vi "Color-Senser-Detrmine-Pro_Test.vi"() -> ()   [LabVIEW 2019]
panel:
  in  "角度":dbl
  out "當前顏色值":T1(array[cluster])
  out "Error Out":errorcluster
  out "對應顏色":enum16{"黃", "紅", "綠", "藍", "黑", "無"}(ring)
  in  "Error In":errorcluster
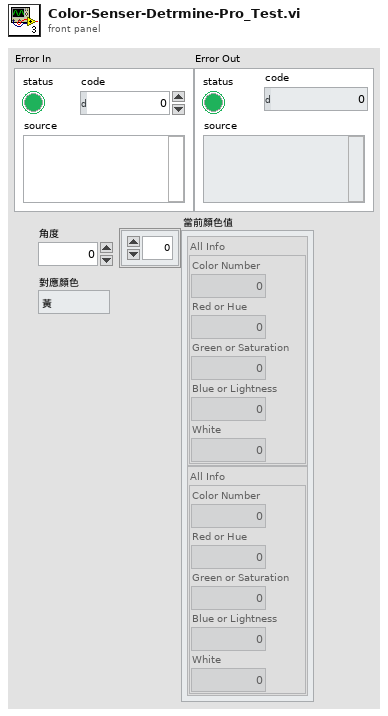
[diagram p1: front panel]
types:
  T1 = cluster{"All Info":cluster{"Color Number":i32, "Red or Hue":i32, "Green or Saturation":i32, "Blue or Lightness":i32, "White":i32}}[]
  T2 = typedef "I2C.lvlib/I2C Reference.ctl" = cluster{"myRIO Reference":T3, "I2C Channels Enum":T7, "I2C Configuration":T8}
  T3 = typedef "myRIO Generic Hardware Reference.ctl" = cluster{"myRIO Model":T4, "myRIO Hardware Reference":T5}
  T4 = typedef "Hardware Version Enum.ctl" = enum16{"Unknown", "myRIO-1900", "myRIO-1950", "roboRIO", "NI ELVIS RIO CM", "ELVIS III"}
  T5 = typedef "myRIO v1.0 Reference.ctl" = cluster{"Generic FPGA Reference":T6, "Allow multiple opens":bool}
  T6 = typedef "Generic FPGA Reference.ctl" = refnum<k20>
  T7 = typedef "I2C Channels Enum.ctl" = enum16{"Not Connected", "A/I2C", "B/I2C", "I2C/I2C"}
  T8 = typedef "I2C.lvlib/I2C Configuration.ctl" = cluster{"I2C Transfer Rate":T9}
  T9 = typedef "I2C.lvlib/I2C Transfer Rate.ctl" = enum16{"Standard mode (100 kbps)", "Fast mode (400 kbps)"}
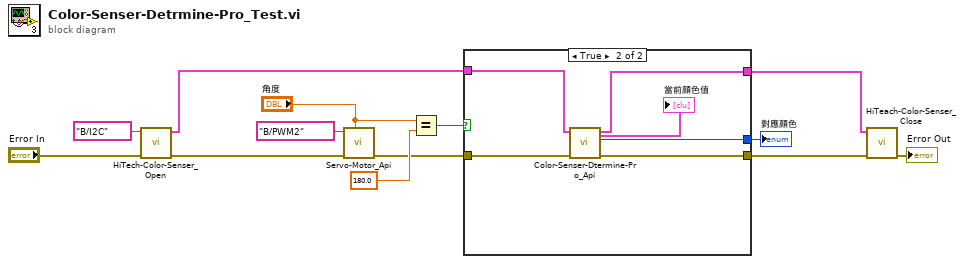
[diagram p0: block diagram]
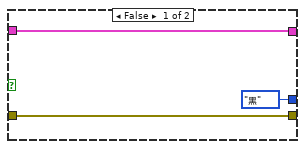
[diagram p2: hidden frame]
diagram:
  n1 = call "HiTech-Color-Senser_Open.vi"("Error In"="Error In", "I2C角位"=tag "B/I2C") -> ("Error Out"=w11:errorcluster, "HiTechnicColorSensorV2 Ref Out"=w9:cluster{"I2C Ref Out":T2})  [unwired: 8 in]
  n2 = call "Servo-Motor_Api.vi"("角度"="角度", "Error In"=w11, "伺服馬達角位"=tag "B/PWM2") -> ("Error Out"=w4:errorcluster)  [unwired: 8 in]
  n3 = Equal?(x="角度", y=180.0) -> (x = y?=w2:bool)
  n4 = case shown="True" w2 {
    tunnel: w4 -> [w15 w18]
    tunnel: [w15 w22] -> w13
    tunnel: [enum16{"黃", "紅", "綠", "藍", "黑"}."黑" ("對應顏色") w21] -> w3
    tunnel: w9 -> [w16 w20]
    tunnel: [w16 w19] -> w8
    frame False {
    }
    frame True {
      n5 = call "Color-Senser-Dtermine-Pro_Api.vi"("Error In"=w18, "HiTechnicColorSensorV2 Ref In"=w20) -> ("Error Out"=w22:errorcluster, "對應顏色"=w21:enum16{"黃", "紅", "綠", "藍", "黑", "無"}, "HiTechnicColorSensorV2 Ref Out"=w19:cluster{"I2C Ref Out":T2}, "當前顏色值"=→"當前顏色值":T1)  [unwired: 4 in, 2 out]
    }
  }
  "對應顏色" <- w3
  n6 = call "HiTeach-Color-Senser_Close.vi"("Error In"=w13, "HiTechnicColorSensorV2 Ref"=w8) -> ("Error Out"=→"Error Out":errorcluster)  [unwired: 9 in]
